vi "ILABR_IsLoaded.vi"(1 "port":u32, 2 "machineName":string, 3 "name":string) -> (0 "status":bool)   [LabVIEW 2009]
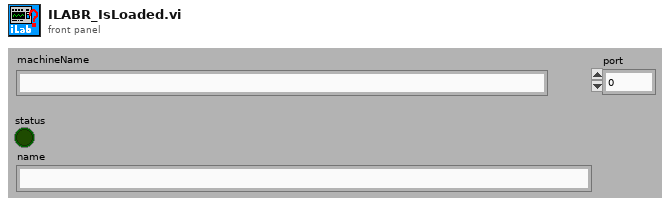
[diagram p1: front panel]
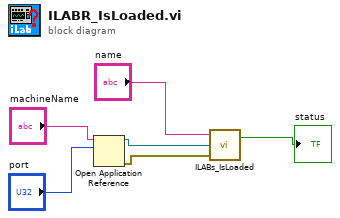
[diagram p0: block diagram]
diagram:
  n1 = Open Application Reference(10:"port", 11:"machineName") -> (0:w6:errorcluster, 3:w5:refnum<vi>)  [unwired: 1 in, 1 out]
  n2 = call "ILABs_IsLoaded.vi"("error in (no error)"=w6, "appRef"=w5, "name"="name") -> ("status"=→"status":bool)  [unwired: 1 out]
